vi "Read Ultrasonic.vi"(11 "ultrasonic name":string) -> (3 "Range":dbl)   [LabVIEW 2014]
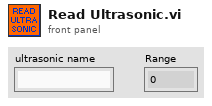
[diagram p1: front panel]
types:
  T1 = typedef "WPI_AnalogChannelDevRef.ctl" = cluster{"DevStatus":errorcluster, "Controller":T2, "Analog Channel":T3}
  T2 = typedef "FPGA_TypedefAnalogModule.ctl" = enum16{"Controller 1"}
  T3 = typedef "FPGA_AIChannel.ctl" = enum8{"AI 0", "AI 1", "AI 2", "AI 3", "AI MXP 0", "AI MXP 1", "AI MXP 2", "AI MXP 3", "Invalid"}
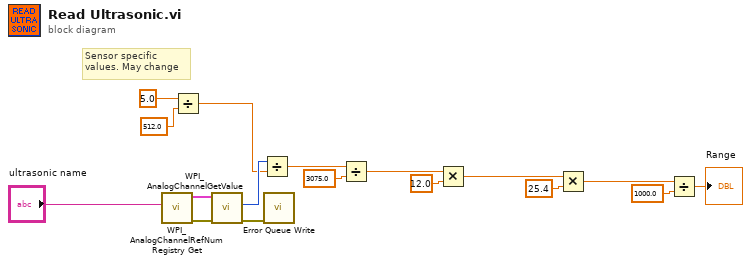
[diagram p0: block diagram]
diagram:
  # "Sensor specific\nvalues. May change"
  n1 = call <vilib>:"WPI_AnalogChannelRefNum Registry Get.vi"("refnum name"="ultrasonic name") -> ("error out"=w2:errorcluster, "AIDeviceRef"=w3:T1)  [unwired: 9 in]
  n2 = Divide(x=5.0, y=512.0) -> (x/y=w13:dbl)
  n3 = call <vilib>:"WPI_AnalogChannelGetValue.vi"("error in (no error)"=w2, "AIDeviceRef"=w3) -> ("error out"=w1:errorcluster, "Value"=w14:i16)  [unwired: 7 in, 1 out]
  n4 = Divide(x=w14, y=w13) -> (x/y=w15:dbl)
  n5 = call "Error Queue Write.vi"("error in (no error)"=w1) -> ()  [unwired: 11 in]
  n6 = Divide(x=w15, y=3075.0) -> (x/y=w7:dbl)
  n7 = Multiply(x=w7, y=12.0) -> (x*y=w9:dbl)
  n8 = Multiply(x=w9, y=25.4) -> (x*y=w11:dbl)
  n9 = Divide(x=w11, y=1000.0) -> (x/y=→"Range":dbl)
